vi "VirtualBench_Protocol_Decoder.vi"(11 "Waveform Graph":waveform(dbl)[](graph)=[{"t0"=timestamp(3765384724.439167 s since 1904-01-01), "dt"=1e-05, "Y"=array[500001 elements], "attributes"=variant("NI_ChannelName"=variant(string "mso/1"), "NI_UnitDescription"=variant(string "Volts"))}]) -> (2 "PassFailed":bool=TRUE, 3 "Result":string)   [LabVIEW 2016]
panel:
  out "Array 3":dbl[](array[numeric])
  out "Array 2":dbl[](array[numeric])
  out "Array":dbl[](array[numeric])
  out "Subwaveform":waveform(dbl)(graph)
  out "Position first transition":dbl
  out "Transition Treshold":dbl
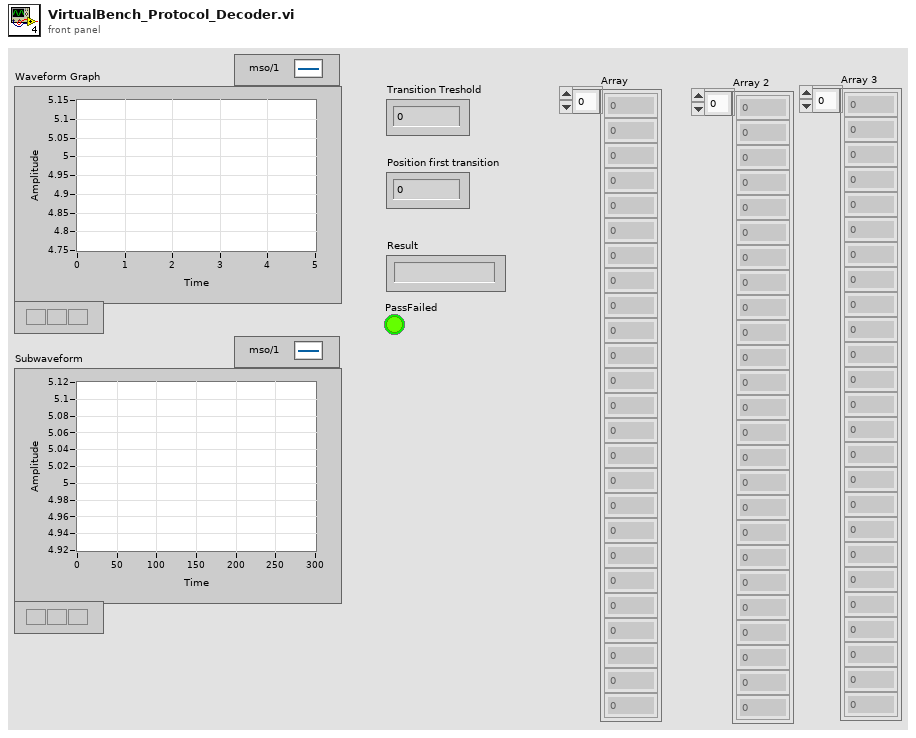
[diagram p1: front panel]
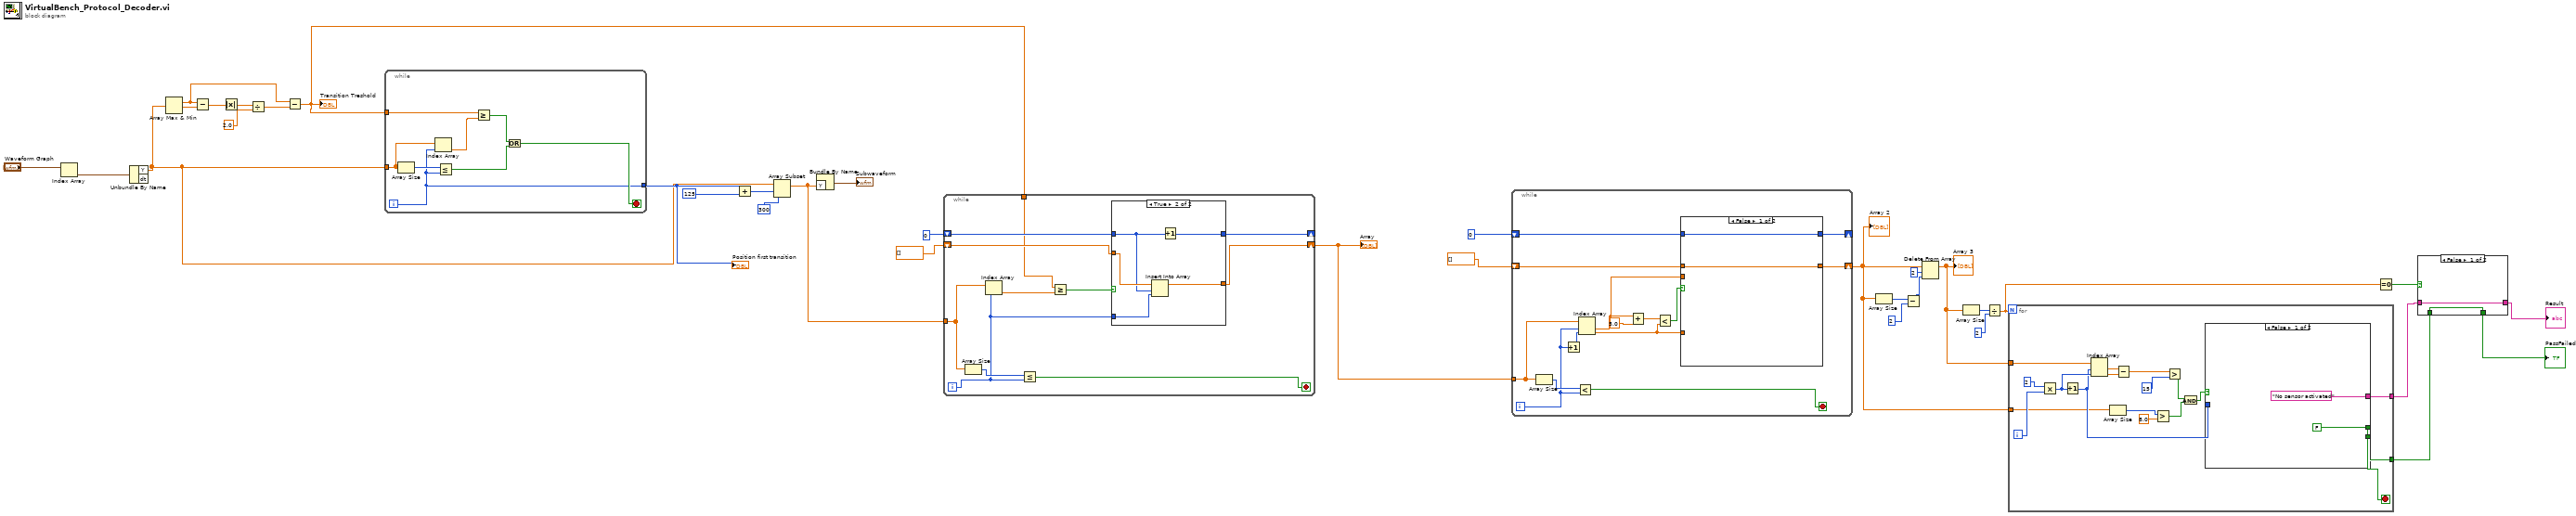
[diagram p0: block diagram]
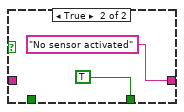
[diagram p2: hidden frame]
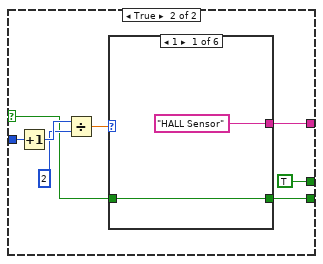
[diagram p3: hidden frame]
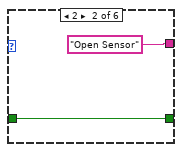
[diagram p4: hidden frame]
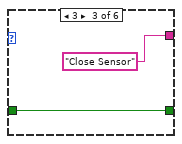
[diagram p5: hidden frame]
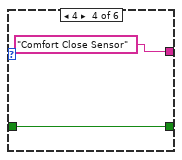
[diagram p6: hidden frame]
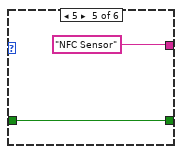
[diagram p7: hidden frame]
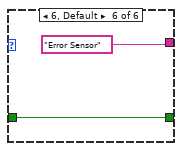
[diagram p8: hidden frame]
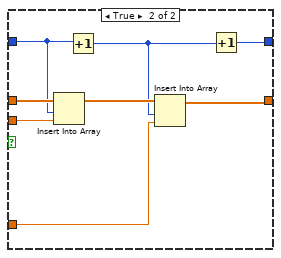
[diagram p9: hidden frame]
diagram:
  n1 = Index Array(array="Waveform Graph") -> (element=w29:waveform(dbl))  [unwired: 1 in]
  n2 = Unbundle By Name(w29) -> ("Y"=w22:dbl[])  [unwired: 1 out]
  n3 = Array Max & Min(array=w22) -> (max value=w33:dbl, min value=w34:dbl)  [unwired: 2 out]
  n4 = Subtract(x=w33, y=w34) -> (x-y=w35:dbl)
  n5 = Absolute Value(x=w35) -> (abs(x)=w32:dbl)
  n6 = Divide(x=w32, y=2.0) -> (x/y=w30:dbl)
  n7 = Subtract(x=w33, y=w30) -> (x-y=w20:dbl)
  "Transition Treshold" <- w20
  n8 = while {
    tunnel: w22 -> [w42]
    tunnel: w20 -> [w37]
    tunnel: [w39] -> w25
    i -> [w39]
    stop <- w40 stop-if-true
    n9 = Array Size(array=w42) -> (size(s)=w43:i32)
    n10 = Index Array(array=w42, index=w39) -> (element=w36:dbl)
    n11 = Less Or Equal?(x=w43, y=w39) -> (x <= y?=w41:bool)
    n12 = Greater Or Equal?(x=w37, y=w36) -> (x >= y?=w38:bool)
    n13 = Or(x=w38, y=w41) -> (x .or. y?=w40:bool)
  }
  "Position first transition" <- w25
  n14 = Add(x=w25, y=125 ("length")) -> (x+y=w23:i32)
  n15 = Array Subset(array=w22, index=w23, length=300) -> (w21:dbl[])
  n16 = Bundle By Name("Y"=w21) -> (→"Subwaveform":waveform(dbl))  [unwired: 1 in]
  n17 = while {
    tunnel: w21 -> [w52]
    tunnel: w20 -> [w45]
    shift-right: [w48] -> _
    shift-left: 0 -> [w49]
    shift-right: [w46] -> w17
    shift-left: dbl[] [] -> [w50]
    i -> [w47]
    stop <- w53 stop-if-true
    n18 = Array Size(array=w52) -> (size(s)=w54:i32)
    n19 = Index Array(array=w52, index=w47) -> (element=w44:dbl)
    n20 = Less Or Equal?(x=w54, y=w47) -> (x <= y?=w53:bool)
    n21 = Greater Or Equal?(x=w45, y=w44) -> (x >= y?=w51:bool)
    n22 = case shown="True" w51 {
      tunnel: w50 -> [w55 w61]
      tunnel: w49 -> [w56 w59]
      tunnel: [w56 w60] -> w48
      tunnel: w47 -> [_ w58]
      tunnel: [w55 w57] -> w46
      frame False {
      }
      frame True {
        n23 = Insert Into Array(array=w61, index=w59, new element=w58) -> (w57:dbl[])
        n24 = Increment(x=w59) -> (x+1=w60:i32)
      }
    }
  }
  "Array" <- w17
  n25 = while {
    tunnel: w17 -> [w73]
    shift-right: [w64] -> _
    shift-left: 0 -> [w65]
    shift-right: [w66] -> w7
    shift-left: dbl[] [] -> [w67]
    i -> [w72]
    stop <- w74 stop-if-true
    n26 = Array Size(array=w73) -> (size(s)=w75:i32)
    n27 = Increment(x=w72) -> (x+1=w71:i32)
    n28 = Less?(x=w75, y=w72) -> (x < y?=w74:bool)
    n29 = Index Array(array=w73, index #1=w72, index #2=w71) -> (element #1=w63:dbl, element #2=w62:dbl)
    n30 = Add(x=w63, y=5.0) -> (x+y=w69:dbl)
    n31 = Less?(x=w69, y=w62) -> (x < y?=w68:bool)
    n32 = case shown="False" w68 {
      tunnel: w67 -> [w76 w85]
      tunnel: [w76 w80] -> w66
      tunnel: w65 -> [w77 w83]
      tunnel: [w77 w84] -> w64
      tunnel: w63 -> [_ w82]
      tunnel: w62 -> [_ w78]
      frame False {
      }
      frame True {
        n33 = Insert Into Array(array=w85, index=w83, new element=w82) -> (w81:dbl[])
        n34 = Increment(x=w83) -> (x+1=w79:i32)
        n35 = Insert Into Array(array=w81, index=w79, new element=w78) -> (w80:dbl[])
        n36 = Increment(x=w79) -> (x+1=w84:i32)
      }
    }
  }
  "Array 2" <- w7
  n37 = Array Size(array=w7) -> (size(s)=w13:i32)
  n38 = Subtract(x=w13, y=2) -> (x-y=w11:i32)
  n39 = Delete From Array(array=w7, length=2, index=w11) -> (array with subset deleted=w10:dbl[])  [unwired: 1 out]
  "Array 3" <- w10
  n40 = Array Size(array=w10) -> (size(s)=w9:i32)
  n41 = Divide(x=w9, y=2) -> (x/y=w6:dbl)
  n42 = for {
    N: w6 -> [_]
    tunnel: w10 -> [w101]
    tunnel: [w94] -> w4
    tunnel: [w92] -> w1
    tunnel: w7 -> [w86]
    i -> [w103]
    stop <- w93 stop-if-true
    n43 = Multiply(x=2, y=w103) -> (x*y=w100:i32)
    n44 = Increment(x=w100) -> (x+1=w95:i32)
    n45 = Index Array(array=w101, index #1=w95, index #2=w100) -> (element #1=w98:dbl, element #2=w99:dbl)
    n46 = Array Size(array=w86) -> (size(s)=w87:i32)
    n47 = Subtract(x=w98, y=w99) -> (x-y=w97:dbl)
    n48 = Greater?(x=w87, y=8.0) -> (0:w90:bool)
    n49 = Greater?(x=w97, y=15) -> (0:w89:bool)
    n50 = And(x=w89, y=w90) -> (x .and. y?=w88:bool)
    n51 = case shown="False" w88 {
      selector: w88 -> [_ w108]
      tunnel: w95 -> [_ w113]
      tunnel: ["No sensor activated" w110] -> w94
      tunnel: [_ w107] -> w93
      tunnel: [FALSE ("Boolean") TRUE ("Boolean")] -> w92
      frame False {
      }
      frame True {
        n52 = Increment(x=w113) -> (x+1=w112:i32)
        n53 = Divide(x=w112, y=2) -> (x/y=w109:dbl)
        n54 = case shown="1" w109 {
          tunnel: ["HALL Sensor" "Open Sensor" "Close Sensor" "Comfort Close Sensor" "NFC Sensor" "Error Sensor"] -> w110
          tunnel: w108 -> [w114 w116 w118 w120 w122 w124]
          tunnel: [w114 w116 w118 w120 w122 w124] -> w107
          frame 1 {
          }
          frame 2 {
          }
          frame 3 {
          }
          frame 4 {
          }
          frame 5 {
          }
          frame 6, Default {
          }
        }
      }
    }
  }
  n55 = Equal To 0?(x=w6) -> (x = 0?=w5:bool)
  n56 = case shown="False" w5 {
    tunnel: w4 -> [w127 _]
    tunnel: [w127 "No sensor activated"] -> w3
    tunnel: [w126 TRUE] -> w2
    tunnel: w1 -> [w126 _]
    frame False {
    }
    frame True {
    }
  }
  "PassFailed" <- w2
  "Result" <- w3
